vi "failure2.vi"() -> ()   [LabVIEW 2018]
panel:
  out "current time 2":timestamp
  in  "current time":timestamp
  in  "Prize":dbl
  in  "Scores":dbl
  in  "Name":string
  out "Table":string[][](table)
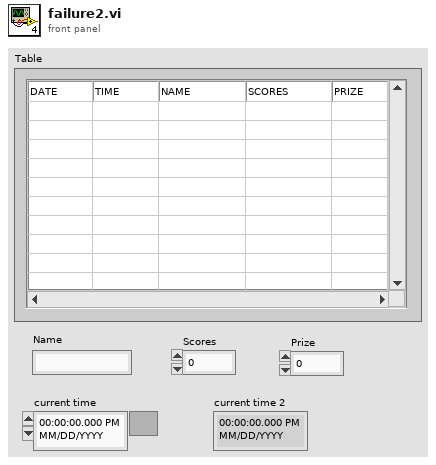
[diagram p1: front panel]
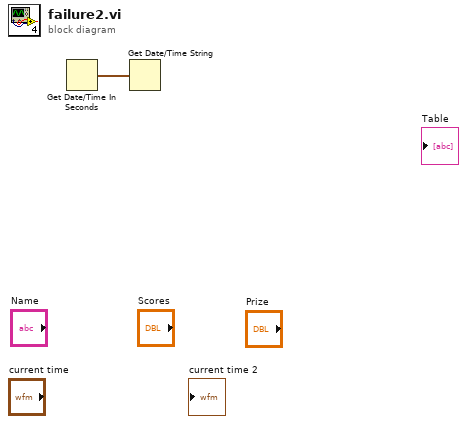
[diagram p0: block diagram]
diagram:
  n1 = Get Date/Time In Seconds() -> (seconds since 1Jan1904=w1:timestamp)
  n2 = Get Date/Time String(seconds (now)=w1) -> ()  [unwired: 2 in, 2 out]
